vi "3_AdvancedDemo_TH260T3.vi"() -> ()   [LabVIEW 2010]
uses:
  Types/TH260_UIThread_Cmds.ctl
  Types/TH260_UIThread_Data.ctl
  Types/TH260_InputChannel.ctl
  <vilib>/Utility/error.llb/DialogType.ctl
  Types/TH260_DataProcThread_QCmds.ctl
  Types/TH260_DataProcThread_QData.ctl
  Types/TH260_VisThread_QCmds.ctl
  Types/TH260_VisThread_QData.ctl
  Types/TH260_VisThread_Data.ctl
  _lib/PQ/TimeHarp260/TH260_InitInfo.ctl
  _lib/PQ/TimeHarp260/th260lib_x86_x64_UIThread.llb/TH260_DllPath_global.vi
  _lib/PQ/TimeHarp260/TH260_LibVersion_global.vi
  _lib/PQ/TimeHarp260/TH260_MeasMode.ctl
  _lib/PQ/TimeHarp260/TH260_TimingMode.ctl
panel:
  in  "Settings":bool=TRUE
  in  "Run continuously":bool caption="Conti."
  in  "Start":bool
  in  "Scale":bool
  out "CountRates":i32[](graph)
  in  "HistoAcqTime":dbl=1.0 caption="Int.Time    s" min=0.1 max=360000.0 step=0.1
  in  "AcqTime":i32=360000000 caption="T3Acq.   ms" min=1 max=360000 step=1
  in  "Binning":i32(ring) caption="Resol.      ps" items=["250", "500", "1000", "2000", "4000", "8000", "16000", "32000", "64000", "128000", "256000", "512000", "1024000", "2048000", "4096000", "8192000", "16384000", "32768000", "65536000", "131072000", "262144000", "524288000"]
  in  "HistoOffset":i32 caption="Offset      ns" min=0 max=500000 step=1
  out "DeltaT":dbl=inf caption="Resol.     ms" format="%.2f"
  in  "BitShift":i32=15 min=0 max=32 step=1
  in  "OvlLevel":u32=65536 caption="Ovl.Level" min=1024 max=65536 step=1024
  in  "StopOvl.":bool=TRUE
  out "TTraceGraph":T1(graph)
  out "HistoGraph":cluster{dbl, "Resol":dbl, "Histos":u32[][]}(graph)
  in  "SyncTrgEdge":i32(ring) caption="Edge" items=["falling", "rising"]
  in  "SyncTrgLevel":i32=-100 caption="Level        mV" min=-1200 max=1200 step=1
  in  "SyncCFDLevel":i32=-100 caption="Level        mV" min=-1200 max=0 step=1
  in  "SyncZeroX":i32=-10 caption="ZeroCr.    mV" min=-40 max=0 step=1
  in  "SyncDivider":i32(ring)=3 caption="Divider" items=["1", "2", "4", "8"]
  in  "SyncOffset":i32 caption="Offset        ps" min=-99999 max=99999 step=1
  in  "Channels":T2[](array[typedef])=[{"Name"="Inp.Chan 1", "Enable"=TRUE, "Offset"=0, "CFDLevel"=50, "ZeroX"=10, "dtcode"=0, "TrgLevel"=-100, "TrgEdge"=0}, {"Name"="Inp.Chan 2", "Enable"=TRUE, "Offset"=0, "CFDLevel"=50, "ZeroX"=10, "dtcode"=0, "TrgLevel"=-100, "TrgEdge"=0}, {"Name"="Inp.Chan 3", "Enable"=TRUE, "Offset"=0, "CFDLevel"=50, "ZeroX"=10, "dtcode"=0, "TrgLevel"=-100, "TrgEdge"=0}, {"Name"="Inp.Chan 4", "Enable"=TRUE, "Offset"=0, "CFDLevel"=50, "ZeroX"=10, "dtcode"=0, "TrgLevel"=-100, "TrgEdge"=0}, {"Name"="Inp.Chan 5", "Enable"=TRUE, "Offset"=0, "CFDLevel"=50, "ZeroX"=10, "dtcode"=0, "TrgLevel"=-100, "TrgEdge"=0}, {"Name"="Inp.Chan 6", "Enable"=TRUE, "Offset"=0, "CFDLevel"=50, "ZeroX"=10, "dtcode"=0, "TrgLevel"=-100, "TrgEdge"=0}, {"Name"="Inp.Chan 7", "Enable"=TRUE, "Offset"=0, "CFDLevel"=50, "ZeroX"=10, "dtcode"=0, "TrgLevel"=-100, "TrgEdge"=0}, {"Name"="Inp.Chan 8", "Enable"=TRUE, "Offset"=0, "CFDLevel"=50, "ZeroX"=10, "dtcode"=0, "TrgLevel"=-100, "TrgEdge"=0}] {"TrgEdge" items=["falling", "rising"]; "TrgLevel" min=-1200 max=1200 step=1; "dtcode" items=["24", "44", "66", "88", "112", "135", "160", "180"]; "ZeroX" min=-40 max=0 step=1; "Offset" min=-99999 max=99999 step=1; "CFDLevel" min=-1200 max=0 step=1}
  out "SyncRate":string="Sync Rate: 0 cps\n"
  out "OverRun":bool caption="Overrun:"
  out "Status":string="Elements in Q: 0"
  # "Histogram"
  # "Time Trace"
  # "Sync"
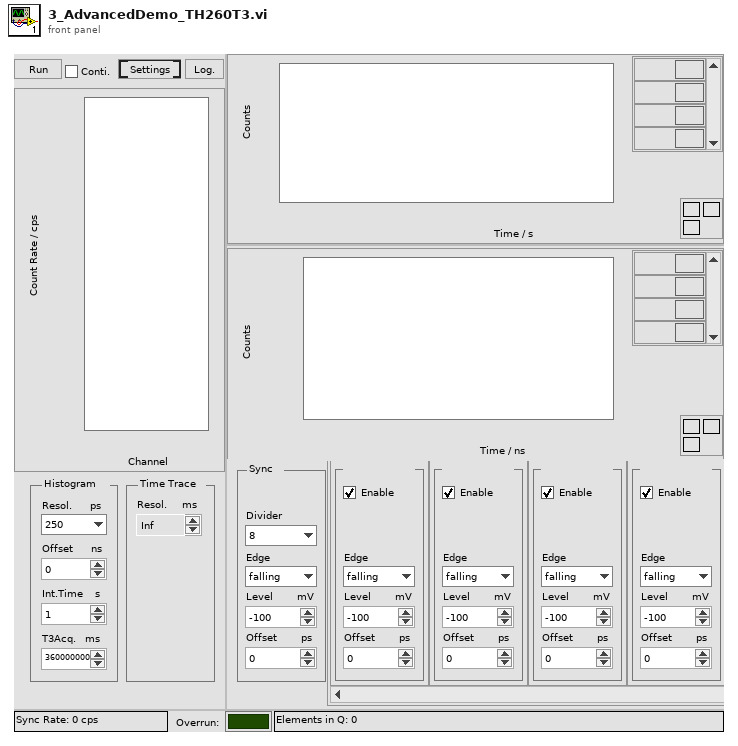
[diagram p1: front panel]
types:
  T1 = cluster{dbl, "Resolution":dbl, "Histogram":u32[][]}
  T2 = typedef "TH260_InputChannel.ctl" = cluster{"Name":string, "Enable":bool, "Offset":i32, "CFDLevel":i32, "ZeroX":i32, "dtcode":i32, "TrgLevel":i32, "TrgEdge":i32}
  T3 = typedef "TH260_DataProcThread_QCmds.ctl" = enum16{"Exit", "Proc", "Init", "SetShift", "SetNumChannels", "SetHistAcqTime"}
  T4 = typedef "TH260_VisThread_Data.ctl" = cluster{"Resol":dbl, "DeltaT":dbl, "NumChannels":i32}
  T5 = typedef "TH260_VisThread_QData.ctl" = cluster{"Histos":u32[][], "Cmd":T6, "TimeTrace":u32[][], "Bin":i32, "Total bin":u64, "Status":string, "Resol":dbl, "DeltaT":dbl, "nChannels":i32}
  T6 = typedef "TH260_VisThread_QCmds.ctl" = enum16{"_none_", "Resol", "nChannels", "DeltaT", "Histo", "TTrace", "Status"}
  T7 = typedef "TH260_DataProcThread_QData.ctl" = cluster{"Cmd":T3, "nActual":i32, "Buffer":u32[], "TickCount":u32, "Param":i32}
  T8 = typedef "TH260_UIThread_Data.ctl" = cluster{"Init Info":T9, "DevIdx":i32, "Channels":T2[], "CurrentChannels":i32[], "AcqTime":i32, "Binning":i32, "HistoOffset":i32, "HistoLen":i32, "StopOvl.":bool, "OvlLevel":u32, "StartMeas":bool, "HistoLength":i32, "Resolution":dbl, "Run cont.":bool, "Status":string, "SyncRate":i32, "BitShift":i32, "HistoAcqTime":dbl, "SyncTrgEdge":i32, "SyncTrgLevel":i32, "SyncCFDLevel":i32, "SyncZeroX":i32, "SyncDivider":i32, "SyncOffset":i32}
  T9 = typedef "TH260_InitInfo.ctl" = cluster{"Library Version":string, "Serial No.":string, "Model":string, "Partnum":string, "Version":string, "features":i32, "nchannels":i32, "Base Resolution":dbl, "Bin Steps":i32}
  T10 = typedef "TH260_UIThread_Cmds.ctl" = enum16{"Idle", "Init", "SetInpChanEnable", "SetInpChanOffset", "SetInpChanCFD", "SetInpChanTrg", "SetInpChanDeadtime", "SetSyncDivider", "SetSyncCFD", "SetSyncTrg", "SetSyncOffset", "SetBinning", "SetHistoOffset", "SetHistoLen", "SetStopOvl", "SetBitShift", "SetHistoAcqTime", "GetRates", "StartMeas", "StopMeas", "AbortMeas", "GetResolution", "GetHisto", "ReadFiFo", "WriteStatus", "Resize", "EnableControls", "DisableControls", "Error", "Exit"}
  T11 = enum8{"Enabled", "Disabled", "Disabled and Grayed Out"}
  T12 = typedef "TH260_TimingMode.ctl" = i32
  T13 = typedef "TH260_MeasMode.ctl" = i32
  T14 = typedef "DialogType.ctl" = u16
  T15 = cluster{"T0":dbl, "dt":dbl, "TimeTrace_out":u32[][]}
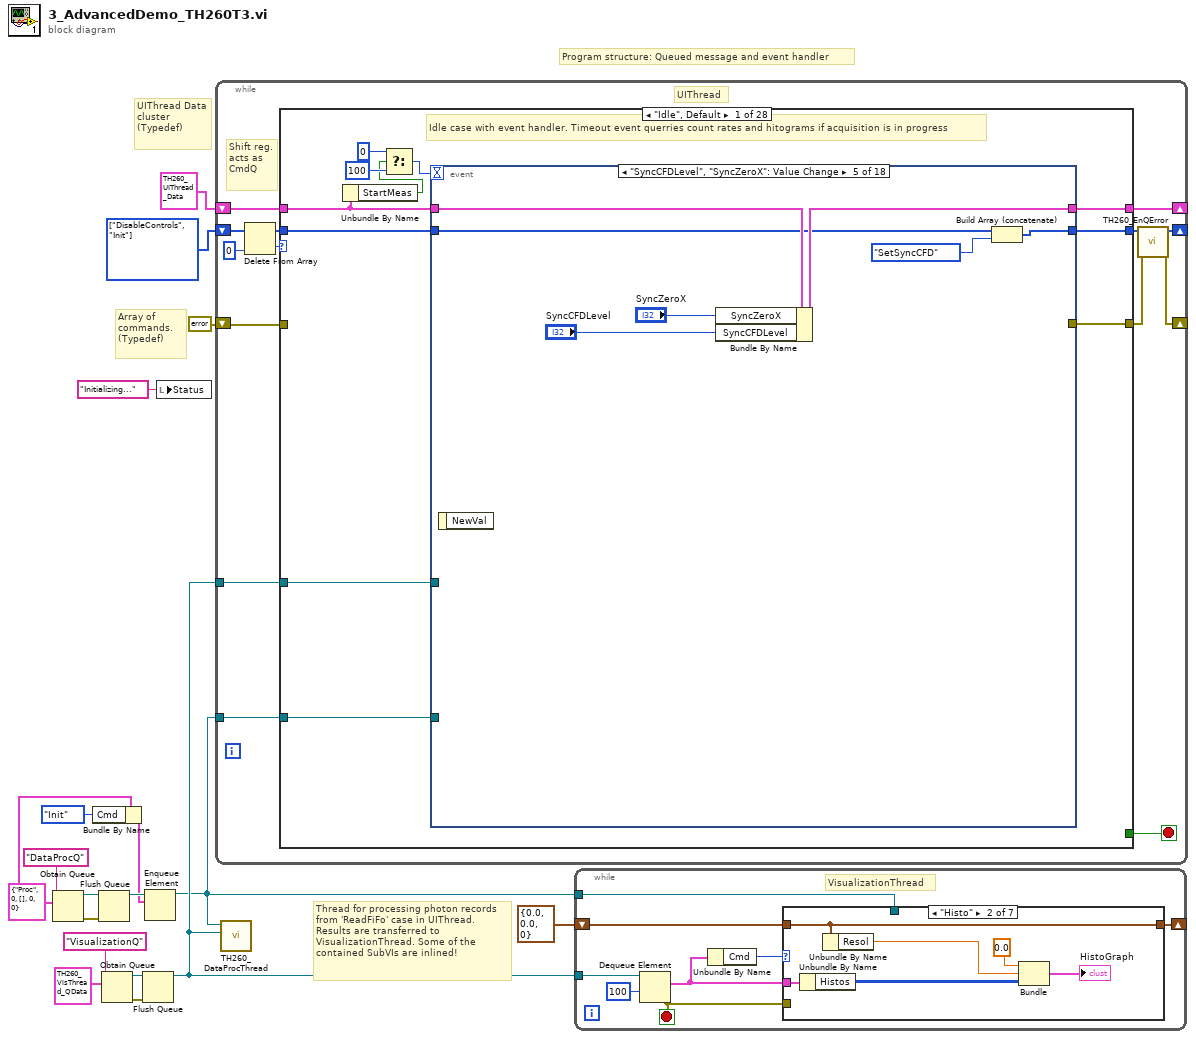
[diagram p0: block diagram]
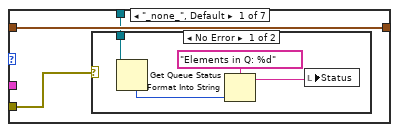
[diagram p2: hidden frame]
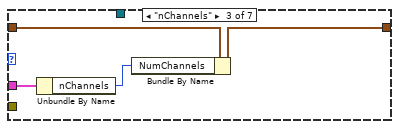
[diagram p4: hidden frame]
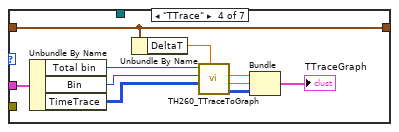
[diagram p5: hidden frame]
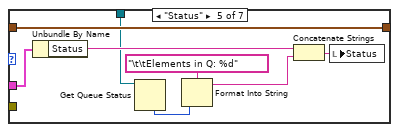
[diagram p6: hidden frame]
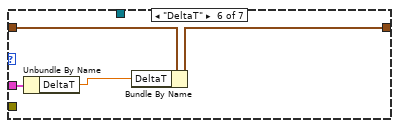
[diagram p7: hidden frame]
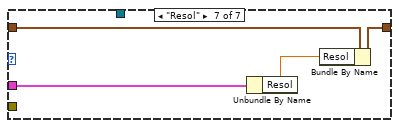
[diagram p8: hidden frame]
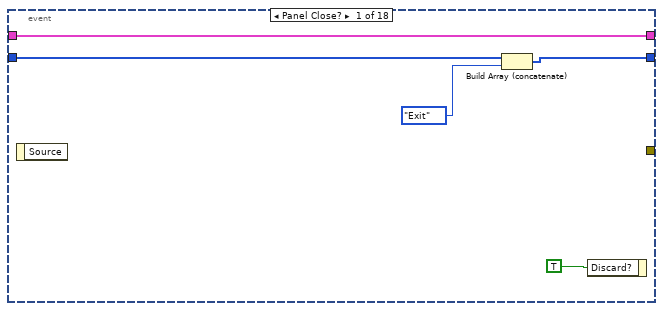
[diagram p9: hidden frame]
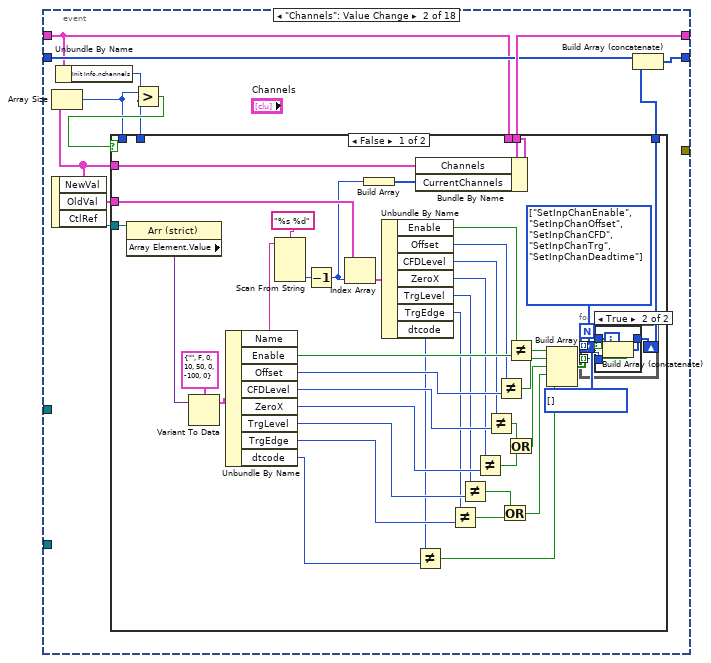
[diagram p10: hidden frame]
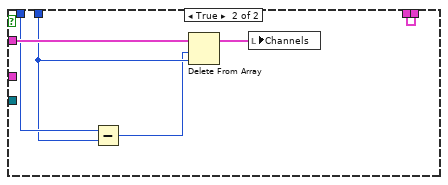
[diagram p12: hidden frame]
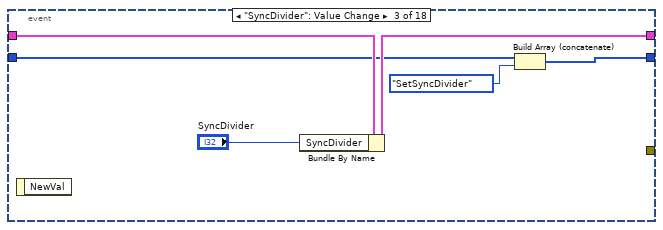
[diagram p13: hidden frame]
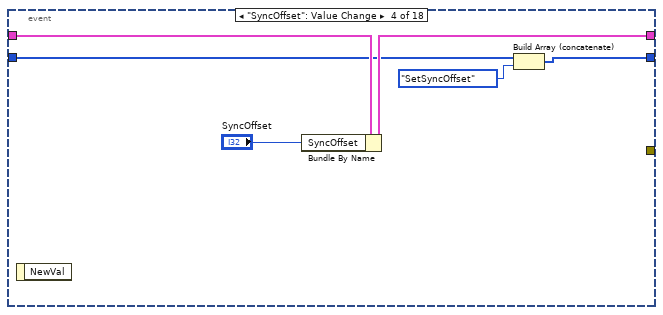
[diagram p14: hidden frame]
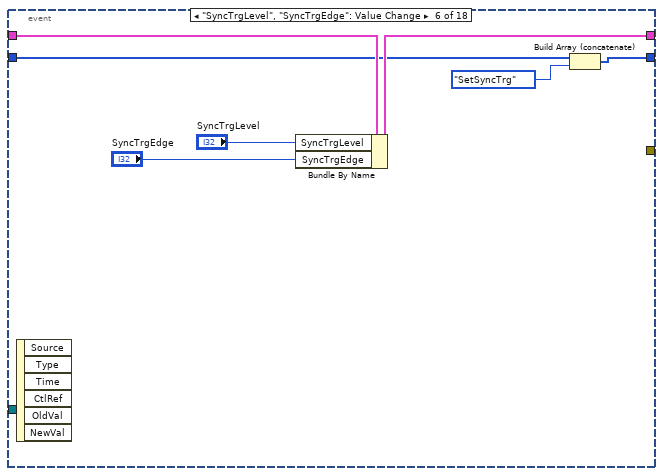
[diagram p15: hidden frame]
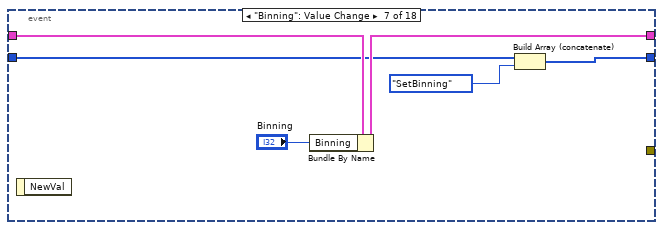
[diagram p16: hidden frame]
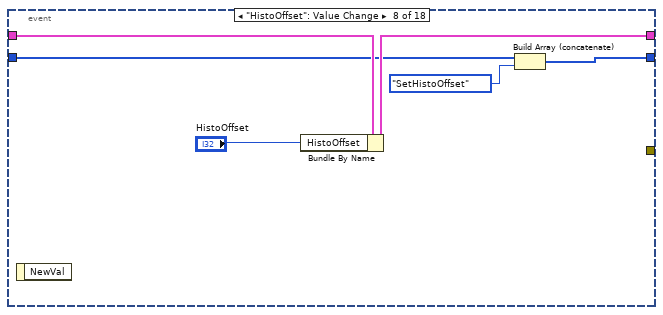
[diagram p17: hidden frame]
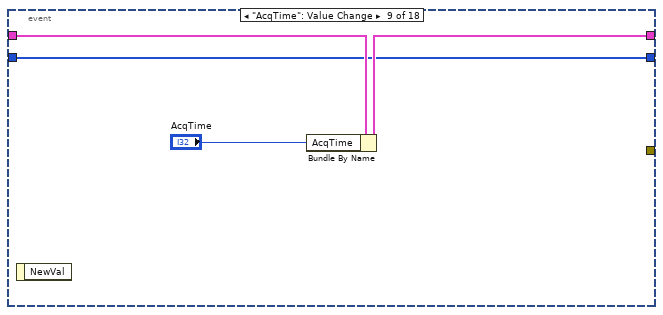
[diagram p18: hidden frame]
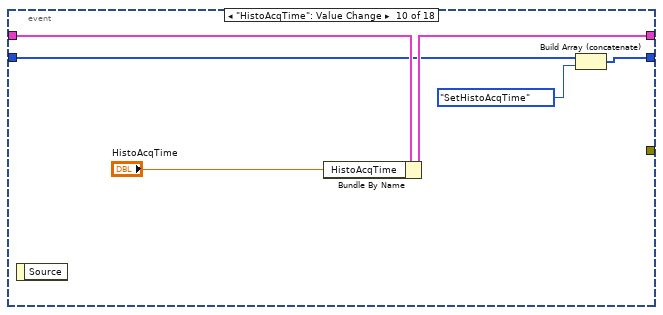
[diagram p19: hidden frame]
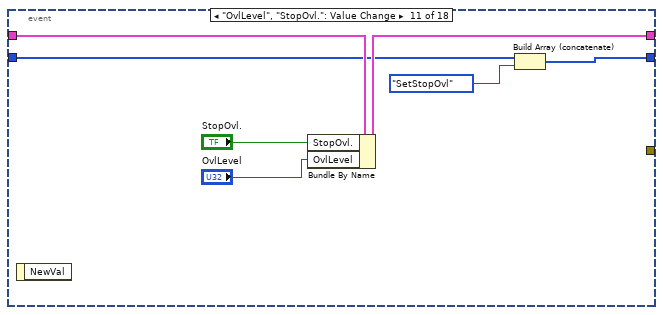
[diagram p20: hidden frame]
diagram:
  w4 = T7 {"Cmd"=enum."Proc", "nActual"=0, "Buffer"=[], "TickCount"=0, "Param"=0} ("MH_DataProcThread_QData")
  w17 = T10[] [enum."DisableControls", enum."Init"] items=["Idle", "Init", "SetInpChanEnable", "SetInpChanOffset", "SetInpChanCFD", "SetInpChanTrg", "SetInpChanDeadtime", "SetSyncDivider", "SetSyncCFD", "SetSyncTrg", "SetSyncOffset", "SetBinning", "SetHistoOffset", "SetHistoLen", "SetStopOvl", "SetBitShift", "SetHistoAcqTime", "GetRates", "StartMeas", "StopMeas", "AbortMeas", "GetResolution", "GetHisto", "ReadFiFo", "WriteStatus", "Resize", "EnableControls", "DisableControls", "Error", "Exit"]
  # "Thread for processing photon records from 'ReadFiFo' case in UIThread. Results are transferred to VisualizationThread. Some of the contained SubVIs are inlined!"
  # "Array of commands.\n(Typedef)"
  # "Program structure: Queued message and event handler"
  # "UIThread Data cluster\n(Typedef)"
  n1 = Obtain Queue(name (unnamed)="DataProcQ", element data type=w4) -> (queue out=w14:refnum<queue>, error out=w13:errorcluster)  [unwired: 3 in, 1 out]
  n2 = Bundle By Name(cluster=w4, "Cmd"=TH260_DataProcThread_QCmds."Init") -> (w2:T7)
  n3 = Flush Queue(queue=w14, error in (no error)=w13) -> (queue out=w5:refnum<queue>)  [unwired: 2 out]
  n4 = Obtain Queue(name (unnamed)="VisualizationQ", element data type=T5 {"Histos"=[], "Cmd"=enum."_none_", "TimeTrace"=[], "Bin"=0, "Total bin"=0, "Status"="", "Resol"=0.0, "DeltaT"=0.0, "nChannels"=0} ("MH_GUIThread_QData")) -> (queue out=w12:refnum<queue>, error out=w11:errorcluster)  [unwired: 3 in, 1 out]
  n5 = Flush Queue(queue=w12, error in (no error)=w11) -> (queue out=w7:refnum<queue>)  [unwired: 2 out]
  n6 = Enqueue Element(queue=w5, element=w2) -> (queue out=w1:refnum<queue>)  [unwired: 2 in, 2 out]
  n7 = local write "Status"("Initializing..." ("Status")) -> ()
  n8 = while {
    shift-right: [w21] -> _
    shift-left: w17 -> [w28]
    shift-right: [w31] -> _
    shift-left: T8 {"Init Info"={"Library Version"="", "Serial No."="", "Model"="", "Partnum"="", "Version"="", "features"=0, "nchannels"=0, "Base Resolution"=0.0, "Bin Steps"=0}, "DevIdx"=0, "Channels"=[], "CurrentChannels"=[], "AcqTime"=1, "Binning"=1, "HistoOffset"=1, "HistoLen"=1024, "StopOvl."=FALSE, "OvlLevel"=1024, "StartMeas"=FALSE, "HistoLength"=0, "Resolution"=0.0, "Run cont."=FALSE, "Status"="", "SyncRate"=0, "BitShift"=0, "HistoAcqTime"=0.0, "SyncTrgEdge"=50, "SyncTrgLevel"=0, "SyncCFDLevel"=-100, "SyncZeroX"=10, "SyncDivider"=1, "SyncOffset"=0} -> [w30]
    shift-right: [w23] -> _
    shift-left: errorcluster {"status"=FALSE, "code"=0, "source"=""} ("error IO") -> [w29]
    tunnel: w1 -> [w20]
    tunnel: w7 -> [w19]
    stop <- w32 stop-if-true
    # "Shift reg.\nacts as\nCmdQ"
    # "UIThread"
    n9 = Delete From Array(array=w28, index=0) -> (deleted portion=w26:T10, array with subset deleted=w25:T10[])  [unwired: 1 in]
    n10 = case shown="\"Idle\", Default" w26 {
      tunnel: [w43 w308 w337 w351 w365 w380 w395 w411 w420 w426 w428 w435 w443 w449 w469 w481 w493 w513 w519 w532 w549 w550 w576 w589 w596 w608 w614 w620] -> w22
      tunnel: [_ _ _ _ _ _ _ _ _ _ _ _ _ _ _ _ _ _ _ _ _ _ _ _ _ _ _ TRUE] -> w32
      tunnel: [w42 w289 w340 w354 w368 w383 w398 w413 w421 w427 w432 w439 w444 w450 w454 w471 w483 w517 w522 w534 w545 w560 w575 w577 w595 w607 w615 w623] -> w31
      tunnel: w30 -> [w39 w294 w340 w354 w368 w383 w398 w413 w421 w427 w432 w439 w444 w450 w454 w471 w484 w517 w523 w535 w546 w560 w575 w577 w595 w607 w615 w623]
      tunnel: [w40 w312 w338 w352 w366 w381 w396 w409 w419 w425 w431 w438 w442 w448 _ _ w492 w516 w525 w537 w547 w555 _ _ _ _ _ w621] -> w24
      tunnel: w29 -> [_ _ _ _ _ _ _ _ _ _ _ _ _ _ _ _ _ _ _ _ _ _ _ _ _ _ w616 _]
      tunnel: w25 -> [w41 w309 w337 w351 w365 w380 w395 w411 w420 w426 w428 w434 w443 w449 w469 w481 w493 w514 w520 w532 w549 w551 w576 w589 w596 w608 _ w620]
      tunnel: w20 -> [w34 w287 _ _ _ _ _ _ _ _ _ _ _ _ w455 w472 _ w510 _ _ _ w552 _ _ _ _ _ w619]
      tunnel: w19 -> [w33 w279 _ _ _ _ _ _ _ _ _ _ _ _ w456 _ _ _ _ _ w542 _ _ _ _ _ _ w618]
      frame "Idle", Default {
        # "Idle case with event handler. Timeout event querries count rates and hitograms if acquisition is in progress"
        n11 = Unbundle By Name(w39) -> ("StartMeas"=w37:bool)
        n12 = Select(t=0, s=w37, f=100) -> (s? t:f=w36:i32)
        n13 = event shown="[4] \"SyncCFDLevel\", \"SyncZeroX\": Value Change" {
          selector: _ -> [_ _ _ _ _ _ _ _ _ _ _ _ _ _ _ _ _ _]
          dyn-events: _ -> [_ _ _ _ _ _ _ _ _ _ _ _ _ _ _ _ _ _]
          timeout: w36 -> [_ _ _ _ _ _ _ _ _ _ _ _ _ _ _ _ _ _]
          tunnel: [w44 w54 w116 w122 w129 w136 w142 w148 w153 w158 w165 w180 w198 w210 w228 w234 w242 w252] -> w43
          tunnel: [w47 w57 w119 w125 w132 w139 w145 w151 w155 w161 w168 w179 w202 w209 w226 w233 w241 w255] -> w42
          tunnel: w39 -> [w47 w53 w120 w126 w133 w140 w146 w152 w156 w162 w169 w179 w203 w207 w227 w233 w241 w255]
          tunnel: w41 -> [w46 w56 w118 w124 w131 w138 w144 w150 w153 w159 w167 w181 w199 w211 w228 w234 w242 w253]
          tunnel: [_ _ _ _ _ _ _ _ _ _ _ w175 _ _ _ _ _ _] -> w40
          tunnel: w34 -> [_ _ _ _ _ _ _ _ _ _ _ _ _ _ _ _ _ _]
          tunnel: w33 -> [_ _ _ _ _ _ _ _ _ _ _ _ _ _ _ _ _ _]
          event Panel Close? {
            n14 = event-data() -> ()  [unwired: 1 in, 1 out]
            n15 = Build Array (concatenate)(w46, TH260_UIThread_Cmds."Exit") -> (w44:T10[])
            n16 = event-data("Discard?"=TRUE) -> ()  [unwired: 1 in, 1 out]
          }
          event "Channels": Value Change {
            n17 = event-data() -> ("NewVal"=w52:T2[], "OldVal"=w58:T2[], "CtlRef"=w59:refnum<vi>)  [unwired: 1 in]
            n18 = Array Size(array=w52) -> (size(s)=w49:i32)
            n19 = Unbundle By Name(w53) -> ("Init Info.nchannels"=w50:i32)
            n20 = Greater?(x=w49, y=w50) -> (0:w51:bool)
            n21 = case shown="False" w51 {
              tunnel: w59 -> [w100 _]
              tunnel: w58 -> [w94 _]
              tunnel: [w77 w114] -> w57
              tunnel: [w75 _] -> w55
              tunnel: w53 -> [w72 w114]
              tunnel: w52 -> [w71 w113]
              tunnel: w50 -> [_ w111]
              tunnel: w49 -> [_ w112]
              frame False {
                w60 = T10[] [] items=["Idle", "Init", "SetInpChanEnable", "SetInpChanOffset", "SetInpChanCFD", "SetInpChanTrg", "SetInpChanDeadtime", "SetSyncDivider", "SetSyncCFD", "SetSyncTrg", "SetSyncOffset", "SetBinning", "SetHistoOffset", "SetHistoLen", "SetStopOvl", "SetBitShift", "SetHistoAcqTime", "GetRates", "StartMeas", "StopMeas", "AbortMeas", "GetResolution", "GetHisto", "ReadFiFo", "WriteStatus", "Resize", "EnableControls", "DisableControls", "Error", "Exit"] ("Array")
                w78 = T10[] [enum."SetInpChanEnable", enum."SetInpChanOffset", enum."SetInpChanCFD", enum."SetInpChanTrg", enum."SetInpChanDeadtime"] items=["Idle", "Init", "SetInpChanEnable", "SetInpChanOffset", "SetInpChanCFD", "SetInpChanTrg", "SetInpChanDeadtime", "SetSyncDivider", "SetSyncCFD", "SetSyncTrg", "SetSyncOffset", "SetBinning", "SetHistoOffset", "SetHistoLen", "SetStopOvl", "SetBitShift", "SetHistoAcqTime", "GetRates", "StartMeas", "StopMeas", "AbortMeas", "GetResolution", "GetHisto", "ReadFiFo", "WriteStatus", "Resize", "EnableControls", "DisableControls", "Error", "Exit"]
                n22 = property class="Arr (strict)"(reference=w100) -> ("Array Element.Value"=w99:variant)  [unwired: 1 in, 2 out]
                n23 = Variant To Data(Variant=w99, type=T2 {"Name"="", "Enable"=FALSE, "Offset"=0, "CFDLevel"=10, "ZeroX"=50, "dtcode"=0, "TrgLevel"=-100, "TrgEdge"=0} ("Channel")) -> (data=w76:cluster{})  [unwired: 1 in, 1 out]
                n24 = Unbundle By Name(w76) -> ("Name"=w97:string, "Enable"=w91:bool, "Offset"=w89:i32, "CFDLevel"=w87:i32, "ZeroX"=w85:i32, "TrgLevel"=w69:i32, "TrgEdge"=w67:i32, "dtcode"=w62:i32)
                n25 = Scan From String(format string="%s %d", input string=w97) -> (output 2=w95:i32)  [unwired: 5 in, 3 out]
                n26 = Decrement(x=w95) -> (x-1=w74:i32)
                n27 = Index Array(array=w94, index=w74) -> (element=w93:T2)
                n28 = Build Array(w74) -> (w73:i32[])
                n29 = Unbundle By Name(w93) -> ("Enable"=w92:bool, "Offset"=w90:i32, "CFDLevel"=w88:i32, "ZeroX"=w86:i32, "TrgLevel"=w70:i32, "TrgEdge"=w68:i32, "dtcode"=w63:i32)
                n30 = Not Equal?(x=w63, y=w62) -> (x != y?=w61:bool)
                n31 = Bundle By Name(cluster=w72, "Channels"=w71, "CurrentChannels"=w73) -> (w77:T8)
                n32 = Not Equal?(x=w68, y=w67) -> (x != y?=w65:bool)
                n33 = Not Equal?(x=w70, y=w69) -> (x != y?=w66:bool)
                n34 = Not Equal?(x=w86, y=w85) -> (x != y?=w80:bool)
                n35 = Not Equal?(x=w88, y=w87) -> (x != y?=w81:bool)
                n36 = Not Equal?(x=w90, y=w89) -> (x != y?=w83:bool)
                n37 = Or(x=w66, y=w65) -> (x .or. y?=w64:bool)
                n38 = Not Equal?(x=w92, y=w91) -> (x != y?=w84:bool)
                n39 = Or(x=w81, y=w80) -> (x .or. y?=w79:bool)
                n40 = Build Array(w84, w83, w79, w64, w61) -> (w82:bool[])
                n41 = for {
                  tunnel: w82 -> [w103] mode=indexing
                  tunnel: w78 -> [w104] mode=indexing
                  shift-right: [w101] -> w75
                  shift-left: w60 -> [w102]
                  n42 = case shown="True" w103 {
                    tunnel: w102 -> [w105 w107]
                    tunnel: w104 -> [_ w106]
                    tunnel: [w105 w108] -> w101
                    frame False {
                    }
                    frame True {
                      n43 = Build Array (concatenate)(w107, w106) -> (w108:T10[])
                    }
                  }
                }
              }
              frame True {
                n44 = Subtract(x=w112, y=w111) -> (x-y=w110:i32)
                n45 = Delete From Array(array=w113, length=w110, index=w111) -> (array with subset deleted=w109:T2[])  [unwired: 1 out]
                n46 = local write "Channels"(w109) -> ()
              }
            }
            n47 = Build Array (concatenate)(w56, w55) -> (w54:T10[])
          }
          event "SyncDivider": Value Change {
            n48 = event-data() -> ()  [unwired: 1 in, 1 out]
            n49 = Bundle By Name(cluster=w120, "SyncDivider"="SyncDivider") -> (w119:T8)
            n50 = Build Array (concatenate)(w118, TH260_UIThread_Cmds."SetSyncDivider") -> (w116:T10[])
          }
          event "SyncOffset": Value Change {
            n51 = event-data() -> ()  [unwired: 1 in, 1 out]
            n52 = Bundle By Name(cluster=w126, "SyncOffset"="SyncOffset") -> (w125:T8)
            n53 = Build Array (concatenate)(w124, TH260_UIThread_Cmds."SetSyncOffset") -> (w122:T10[])
          }
          event "SyncCFDLevel", "SyncZeroX": Value Change {
            n54 = event-data() -> ()  [unwired: 1 in, 1 out]
            n55 = Bundle By Name(cluster=w133, "SyncZeroX"="SyncZeroX", "SyncCFDLevel"="SyncCFDLevel") -> (w132:T8)
            n56 = Build Array (concatenate)(w131, TH260_UIThread_Cmds."SetSyncCFD") -> (w129:T10[])
          }
          event "SyncTrgLevel", "SyncTrgEdge": Value Change {
            n57 = event-data() -> ()  [unwired: 1 in, 6 out]
            n58 = Bundle By Name(cluster=w140, "SyncTrgLevel"="SyncTrgLevel", "SyncTrgEdge"="SyncTrgEdge") -> (w139:T8)
            n59 = Build Array (concatenate)(w138, TH260_UIThread_Cmds."SetSyncTrg") -> (w136:T10[])
          }
          event "Binning": Value Change {
            n60 = event-data() -> ()  [unwired: 1 in, 1 out]
            n61 = Bundle By Name(cluster=w146, "Binning"="Binning") -> (w145:T8)
            n62 = Build Array (concatenate)(w144, TH260_UIThread_Cmds."SetBinning") -> (w142:T10[])
          }
          event "HistoOffset": Value Change {
            n63 = event-data() -> ()  [unwired: 1 in, 1 out]
            n64 = Bundle By Name(cluster=w152, "HistoOffset"="HistoOffset") -> (w151:T8)
            n65 = Build Array (concatenate)(w150, TH260_UIThread_Cmds."SetHistoOffset") -> (w148:T10[])
          }
          event "AcqTime": Value Change {
            n66 = event-data() -> ()  [unwired: 1 in, 1 out]
            n67 = Bundle By Name(cluster=w156, "AcqTime"="AcqTime") -> (w155:T8)
          }
          event "HistoAcqTime": Value Change {
            n68 = event-data() -> ()  [unwired: 1 in, 1 out]
            n69 = Bundle By Name(cluster=w162, "HistoAcqTime"="HistoAcqTime") -> (w161:T8)
            n70 = Build Array (concatenate)(w159, TH260_UIThread_Cmds."SetHistoAcqTime") -> (w158:T10[])
          }
          event "OvlLevel", "StopOvl.": Value Change {
            n71 = event-data() -> ()  [unwired: 1 in, 1 out]
            n72 = Bundle By Name(cluster=w169, "StopOvl."="StopOvl.", "OvlLevel"="OvlLevel") -> (w168:T8)
            n73 = Build Array (concatenate)(w167, TH260_UIThread_Cmds."SetStopOvl") -> (w165:T10[])
          }
          event Timeout {
            n74 = event-data() -> ()  [unwired: 1 in, 1 out]
            n75 = Unbundle By Name(w179) -> ("DevIdx"=w177:i32, "StartMeas"=w178:bool, "BitShift"=w174:i32, "SyncRate"=w173:i32)
            n76 = case shown="True" w178 {
              tunnel: w177 -> [_ w197]
              tunnel: [_ w195] -> w176
              tunnel: [_ w192] -> w175
              frame False {
              }
              frame True {
                w193 = T10[] [enum."ReadFiFo"] items=["Idle", "Init", "SetInpChanEnable", "SetInpChanOffset", "SetInpChanCFD", "SetInpChanTrg", "SetInpChanDeadtime", "SetSyncDivider", "SetSyncCFD", "SetSyncTrg", "SetSyncOffset", "SetBinning", "SetHistoOffset", "SetHistoLen", "SetStopOvl", "SetBitShift", "SetHistoAcqTime", "GetRates", "StartMeas", "StopMeas", "AbortMeas", "GetResolution", "GetHisto", "ReadFiFo", "WriteStatus", "Resize", "EnableControls", "DisableControls", "Error", "Exit"]
                w194 = T10[] [enum."StopMeas"] items=["Idle", "Init", "SetInpChanEnable", "SetInpChanOffset", "SetInpChanCFD", "SetInpChanTrg", "SetInpChanDeadtime", "SetSyncDivider", "SetSyncCFD", "SetSyncTrg", "SetSyncOffset", "SetBinning", "SetHistoOffset", "SetHistoLen", "SetStopOvl", "SetBitShift", "SetHistoAcqTime", "GetRates", "StartMeas", "StopMeas", "AbortMeas", "GetResolution", "GetHisto", "ReadFiFo", "WriteStatus", "Resize", "EnableControls", "DisableControls", "Error", "Exit"]
                n77 = call "TH260_CTCStatus.vi"("devidx"=w197) -> ("error out"=w192:errorcluster, "ctcstatus"=w196:i32)  [unwired: 8 in, 1 out]
                n78 = Not Equal To 0?(x=w196) -> (x != 0?=w191:bool)
                n79 = Select(t=w194, s=w191, f=w193) -> (s? t:f=w195:T10[])
              }
            }
            n80 = call "CalcRate.vi"("Refresh(ms)"=u32 100) -> ("updated?"=w171:bool)  [unwired: 8 in, 2 out]
            n81 = case shown="True" w171 {
              tunnel: w174 -> [_ w184]
              tunnel: w173 -> [_ w183]
              tunnel: [_ TH260_UIThread_Cmds."GetRates"] -> w172
              frame False {
              }
              frame True {
                n82 = To Double Precision Float(number=w183) -> (double precision float=w188:dbl)
                n83 = To Double Precision Float(number=w184) -> (double precision float=w189:dbl)
                n84 = Power Of 2(x=w189) -> (2^x=w187:dbl)
                n85 = Multiply(x=w187, y=1000.0) -> (x*y=w186:dbl)
                n86 = Divide(x=w186, y=w188) -> (x/y=w190:dbl)
                n87 = local write "DeltaT"(w190) -> ()
              }
            }
            n88 = Build Array (concatenate)(w181, w176, w172) -> (w180:T10[])
          }
          event "BitShift": Value Change {
            n89 = event-data() -> ()  [unwired: 1 in, 1 out]
            n90 = Bundle By Name(cluster=w203, "BitShift"="BitShift") -> (w202:T8)
            n91 = Build Array (concatenate)(w199, TH260_UIThread_Cmds."SetBitShift") -> (w198:T10[])
          }
          event "Start": Value Change {
            n92 = event-data() -> ()  [unwired: 1 in, 1 out]
            n93 = Unbundle By Name(w207) -> ("SyncRate"=w206:i32)
            n94 = Greater Or Equal?(x=w206, y=10) -> (x >= y?=w204:bool)
            n95 = case shown="True" w204 {
              selector: w204 -> [w213 _]
              tunnel: w211 -> [w215 w224]
              tunnel: [w215 w222] -> w210
              tunnel: [w214 w221] -> w209
              tunnel: "Start" -> [_ w220]
              tunnel: w207 -> [w214 w216]
              frame False {
                n96 = local write "Start"(w213) -> ()
                n97 = One Button Dialog(message="SyncRate too low!!!" ("Status")) -> ()  [unwired: 1 in, 1 out]
              }
              frame True {
                w219 = T10[] [enum."SetBitShift", enum."SetHistoAcqTime", enum."StartMeas"] items=["Idle", "Init", "SetInpChanEnable", "SetInpChanOffset", "SetInpChanCFD", "SetInpChanTrg", "SetInpChanDeadtime", "SetSyncDivider", "SetSyncCFD", "SetSyncTrg", "SetSyncOffset", "SetBinning", "SetHistoOffset", "SetHistoLen", "SetStopOvl", "SetBitShift", "SetHistoAcqTime", "GetRates", "StartMeas", "StopMeas", "AbortMeas", "GetResolution", "GetHisto", "ReadFiFo", "WriteStatus", "Resize", "EnableControls", "DisableControls", "Error", "Exit"]
                n98 = Bundle By Name(cluster=w216, "StartMeas"=w220) -> (w221:T8)
                n99 = Build Array(TH260_UIThread_Cmds."AbortMeas") -> (w217:T10[])
                n100 = Select(t=w219, s=w220, f=w217) -> (s? t:f=w223:T10[])
                n101 = Build Array (concatenate)(w224, w223) -> (w222:T10[])
              }
            }
          }
          event "Run continuously": Value Change {
            n102 = event-data() -> ()  [unwired: 1 in, 1 out]
            n103 = Bundle By Name(cluster=w227, "Run cont."="Run continuously") -> (w226:T8)
          }
          event "Scale": Value Change {
            n104 = event-data() -> ()  [unwired: 1 in, 1 out]
            n105 = Select(t=u8 0 ("Y Scale.Mapping Mode"), s="Scale", f=u8 1 ("Y Scale.Mapping Mode")) -> (s? t:f=w229:u8)
            n106 = property on="HistoGraph" class="WFGraph (strict)"("YScale.Mapping Mode"=w229) -> ()  [unwired: 2 in, 2 out]
          }
          event "Settings": Value Change {
            n107 = event-data() -> ()  [unwired: 1 in, 1 out]
            n108 = property on="Splitter" class="Splitter"() -> ("Position"=w240:i32)  [unwired: 2 in, 2 out]
            n109 = Select(t=250 ("PosT"), s="Settings", f=0 ("PosF")) -> (s? t:f=w237:i32)
            n110 = Subtract(x=w240, y=w237) -> (x-y=w236:i32)
            n111 = while {
              shift-right: [w251] -> _
              shift-left: w236 -> [w244]
              i -> [w250]
              stop <- w247 stop-if-true
              n112 = property on="Splitter 4" class="Splitter"("Position"=w244) -> (error out=w243:errorcluster)  [unwired: 2 in, 1 out]
              n113 = Greater Or Equal?(x=w250, y=10) -> (x >= y?=w248:bool)
              n114 = Decrement(x=w244) -> (x-1=w251:i32)
              n115 = Unbundle(w243) -> ("status"=w246:bool)  [unwired: 2 out]
              n116 = Not(x=w246) -> (.not. x?=w245:bool)
              n117 = Or(x=w245, y=w248) -> (x .or. y?=w247:bool)
            }
          }
          event Panel Resize {
            n118 = event-data() -> ()  [unwired: 1 in, 1 out]
            n119 = Build Array (concatenate)(w253, TH260_UIThread_Cmds."Resize") -> (w252:T10[])
          }
        }
      }
      frame "Init" {
        w265 = -100 ("SyncTrgLevel")
        w266 = 0 ("SyncTrgEdge")
        w268 = T12 0 items=["Hires", "Lowres"]  # TimingMode
        w269 = T13 3 items=["Histo"=0, "T2"=2, "T3"=3]  # MeasMode
        w277 = 1.0 ("HistoAcqTime")
        w278 = 15 ("Value (Signaling)")
        w296 = FALSE ("Run cont.")
        w298 = FALSE ("StartMeas")
        w299 = u32 100000 ("OvlLevel")
        w300 = TRUE ("StopOvl.")
        w301 = 360000000 ("AcqTime")
        w302 = 0 ("HistoOffset")
        w303 = 0 ("Binning")
        w304 = -100 ("SyncLevel")
        w305 = -10 ("SyncZeroX")
        w306 = 0 ("SyncOffset")
        w307 = 3 ("SyncDivider")
        # "100 x 60 x 60 x 1000 = 100 h"
        # "Init all FP controls and corresponding copy in UIThread Data cluster"
        # "EnQ list of commands"
        # "Array with Inp.Chan."
        # "Initialization: 1. Init HW -> get # of channels -> make array for Inp.Channels\n2. Init all FP controls and corresponding fields in UIThread Data cluster\n3. EnQ list of commands for further initialization"
        n120 = call <vilib>:"Error Cluster From Error Code.vi"("is warning? (False)"=FALSE, "show call chain? (False)"=TRUE, "error message (\"\")"="DLL not found!" ("error message (\"\")"), "error code (0)"=5000) -> ("error out"=w271:errorcluster)  [unwired: 5 in]
        n121 = call "GetDLLPath.vi"("DllName_32bit"="TH260Lib.dll" ("name or relative path"), "DllName_64bit"="TH260Lib64.dll" ("name or relative path")) -> ("file exists?"=w273:bool, "DLLPath"=w274:path)  [unwired: 8 in]
        n122 = global write "TH260_DllPath_global.vi" "DllPath"(w274) -> ()
        n123 = Select(t=errorcluster {"status"=FALSE, "code"=0, "source"=""} ("error IO"), s=w273, f=w271) -> (s? t:f=w290:errorcluster)
        n124 = global read "TH260_LibVersion_global.vi" "Library Version"() -> (w270:string)
        n125 = property on="Settings" class="Bool (strict)"("Val(Sgnl)"=TRUE ("Value (Signaling)")) -> ()  [unwired: 2 in, 2 out]
        n126 = property on="Scale" class="Bool (strict)"("Val(Sgnl)"=FALSE ("Value (Signaling)")) -> ()  [unwired: 2 in, 2 out]
        n127 = call "InitTH260_UIThread.vi"("error in (no error)"=w290, "MeasMode"=w269, "TimingMode"=w268, "Library Version"=w270) -> ("error out"=w312:errorcluster, "Init Info"=w264:T9, "DevIdx"=w314:i32)  [unwired: 5 in]
        n128 = Unbundle By Name(w264) -> ("Model"=w263:string)
        n129 = local write "SyncDivider"(w307) -> ()
        n130 = local write "SyncOffset"(w306) -> ()
        n131 = local write "SyncZeroX"(w305) -> ()
        n132 = local write "SyncCFDLevel"(w304) -> ()
        n133 = local write "SyncTrgEdge"(w266) -> ()
        n134 = local write "SyncTrgLevel"(w265) -> ()
        n135 = Bundle By Name(cluster=w294, "DevIdx"=w314, "Status"="Initialized!", "Init Info"=w264) -> (w293:T8)
        n136 = Unbundle By Name(w293) -> ("Init Info.Bin Steps"=w292:i32, "Init Info.Base Resolution"=w267:dbl, "Init Info.nchannels"=w280:i32)
        n137 = for {
          N: w280 -> [_]
          tunnel: T2 {"Name"="", "Enable"=FALSE, "Offset"=0, "CFDLevel"=10, "ZeroX"=50, "dtcode"=0, "TrgLevel"=-100, "TrgEdge"=0} ("Channel") -> [w333]
          tunnel: [w332] -> w311 mode=indexing
          tunnel: [w322] -> w310 mode=indexing
          i -> [w322]
          # "Init values for Inp. Channels"
          n138 = Increment(x=w322) -> (x+1=w325:i32)
          n139 = Format Into String(format string="Ch.%d", w325) -> (resulting string=w323:string)  [unwired: 2 in, 1 out]
          n140 = Format Into String(format string="Inp.Chan %d", w325) -> (resulting string=w330:string)  [unwired: 2 in, 1 out]
          n141 = property on="HistoGraph" class="WFGraph (strict)"("Active Plot"=w322, "Plot.Plot Name"=w323) -> ()  [unwired: 2 in, 2 out]
          n142 = Bundle By Name(cluster=w333, "Name"=w330, "Enable"=TRUE, "Offset"=0, "CFDLevel"=-100 ("CFDZeroX"), "ZeroX"=-10 ("CFDLevel"), "dtcode"=0, "TrgLevel"=-100, "TrgEdge"=0) -> (w332:T2)
          n143 = property on="TTraceGraph" class="WFGraph (strict)"("Active Plot"=w322, "Plot.Plot Name"=w323) -> ()  [unwired: 2 in, 2 out]
        }
        n144 = Bundle By Name(cluster=T5 {"Histos"=[], "Cmd"=enum."_none_", "TimeTrace"=[], "Bin"=0, "Total bin"=0, "Status"="", "Resol"=0.0, "DeltaT"=0.0, "nChannels"=0} ("MH_GUIThread_QData"), "Cmd"=TH260_VisThread_QCmds."nChannels", "nChannels"=w280) -> (w282:T5)
        n145 = call "TH260_CalcBinningValues.vi"("BaseRes"=w267, "Bin Steps"=w292) -> ("BinningValues"=w297:cluster{"String":string, "Value":i32}[])  [unwired: 9 in]
        n146 = property on="Binning" class="Ring (strict)"("StringsAndValues[]"=w297) -> ()  [unwired: 2 in, 2 out]
        n147 = Bundle By Name(cluster=T7 {"Cmd"=enum."Proc", "nActual"=0, "Buffer"=[], "TickCount"=0, "Param"=0} ("MH_DataProcThread_QData"), "Param"=w280, "Cmd"=TH260_DataProcThread_QCmds."SetNumChannels") -> (w286:T7)
        n148 = Enqueue Element(queue=w279, element=w282) -> ()  [unwired: 2 in, 3 out]
        n149 = Enqueue Element(queue=w287, element=w286) -> ()  [unwired: 2 in, 3 out]
        n150 = local write "Channels"(w311) -> ()
        n151 = Bundle By Name(cluster=w293, "Channels"=w311, "CurrentChannels"=w310, "SyncDivider"=w307, "SyncOffset"=w306, "SyncZeroX"=w305, "SyncCFDLevel"=w304, "SyncTrgEdge"=w266, "SyncTrgLevel"=w265, "Binning"=w303, "HistoOffset"=w302, "AcqTime"=w301, "StopOvl."=w300, "OvlLevel"=w299, "StartMeas"=w298, "Run cont."=w296, "BitShift"=w278, "HistoAcqTime"=w277) -> (w289:T8)
        n152 = case shown="\"TimeHarp 260 P\"" w263 {
          tunnel: [FALSE TRUE] -> w262
          tunnel: [w315 w317] -> w260
          frame Default {
            w315 = T10[] [enum."SetSyncDivider", enum."SetSyncOffset", enum."SetSyncTrg", enum."SetInpChanEnable", enum."SetInpChanOffset", enum."SetInpChanTrg", enum."SetBinning", enum."SetHistoOffset", enum."Resize", enum."EnableControls", enum."GetRates", enum."SetBitShift", enum."SetHistoAcqTime", enum."WriteStatus"] items=["Idle", "Init", "SetInpChanEnable", "SetInpChanOffset", "SetInpChanCFD", "SetInpChanTrg", "SetInpChanDeadtime", "SetSyncDivider", "SetSyncCFD", "SetSyncTrg", "SetSyncOffset", "SetBinning", "SetHistoOffset", "SetHistoLen", "SetStopOvl", "SetBitShift", "SetHistoAcqTime", "GetRates", "StartMeas", "StopMeas", "AbortMeas", "GetResolution", "GetHisto", "ReadFiFo", "WriteStatus", "Resize", "EnableControls", "DisableControls", "Error", "Exit"]
          }
          frame "TimeHarp 260 P" {
            w317 = T10[] [enum."SetSyncDivider", enum."SetSyncOffset", enum."SetSyncCFD", enum."SetInpChanEnable", enum."SetInpChanOffset", enum."SetInpChanCFD", enum."SetInpChanDeadtime", enum."SetBinning", enum."SetHistoOffset", enum."Resize", enum."EnableControls", enum."GetRates", enum."SetBitShift", enum."SetHistoAcqTime", enum."WriteStatus"] items=["Idle", "Init", "SetInpChanEnable", "SetInpChanOffset", "SetInpChanCFD", "SetInpChanTrg", "SetInpChanDeadtime", "SetSyncDivider", "SetSyncCFD", "SetSyncTrg", "SetSyncOffset", "SetBinning", "SetHistoOffset", "SetHistoLen", "SetStopOvl", "SetBitShift", "SetHistoAcqTime", "GetRates", "StartMeas", "StopMeas", "AbortMeas", "GetResolution", "GetHisto", "ReadFiFo", "WriteStatus", "Resize", "EnableControls", "DisableControls", "Error", "Exit"]
          }
        }
        n153 = Not(x=w262) -> (.not. x?=w261:bool)
        n154 = property on="dtcode" class="Ring (strict)"("Visible"=w262) -> ()  [unwired: 2 in, 2 out]
        n155 = property on="SyncZeroX" class="DigNum (strict)"("Visible"=w262) -> ()  [unwired: 2 in, 2 out]
        n156 = property on="SyncCFDLevel" class="DigNum (strict)"("Visible"=w262) -> ()  [unwired: 2 in, 2 out]
        n157 = local write "Binning"(w303) -> ()
        n158 = local write "HistoOffset"(w302) -> ()
        n159 = local write "StopOvl."(w300) -> ()
        n160 = local write "OvlLevel"(w299) -> ()
        n161 = local write "Start"(w298) -> ()
        n162 = local write "Run continuously"(w296) -> ()
        n163 = local write "BitShift"(w278) -> ()
        n164 = local write "AcqTime"(w301) -> ()
        n165 = local write "HistoAcqTime"(w277) -> ()
        n166 = property on="CFDLevel" class="DigNum (strict)"("Visible"=w262) -> ()  [unwired: 2 in, 2 out]
        n167 = property on="ZeroX" class="DigNum (strict)"("Visible"=w262) -> ()  [unwired: 2 in, 2 out]
        n168 = property on="SyncTrgLevel" class="DigNum (strict)"("Visible"=w261) -> ()  [unwired: 2 in, 2 out]
        n169 = property on="SyncTrgEdge" class="Ring (strict)"("Visible"=w261) -> ()  [unwired: 2 in, 2 out]
        n170 = property on="TrgLevel" class="DigNum (strict)"("Visible"=w261) -> ()  [unwired: 2 in, 2 out]
        n171 = property on="TrgEdge" class="Ring (strict)"("Visible"=w261) -> ()  [unwired: 2 in, 2 out]
        n172 = Build Array (concatenate)(w309, w260) -> (w308:T10[])
      }
      frame "SetInpChanEnable" {
        n173 = Unbundle By Name(w340) -> ("DevIdx"=w339:i32, "Channels"=w334:T2[], "CurrentChannels"=w335:i32[])
        n174 = for {
          tunnel: w339 -> [w347]
          shift-right: [w346] -> w338
          shift-left: errorcluster {"status"=FALSE, "code"=0, "source"=""} ("error out") -> [w345]
          tunnel: w335 -> [w341] mode=indexing
          tunnel: w334 -> [w344]
          n175 = Index Array(array=w344, index=w341) -> (element=w343:T2)
          n176 = Unbundle By Name(w343) -> ("Enable"=w342:bool)
          n177 = call "TH260_SetInputChannelEnable.vi"("error in (no error)"=w345, "enable"=w342, "channel"=w341, "devidx"=w347) -> ("error out"=w346:errorcluster)  [unwired: 6 in, 1 out]
        }
      }
      frame "SetInpChanOffset" {
        n178 = Unbundle By Name(w354) -> ("DevIdx"=w353:i32, "Channels"=w348:T2[], "CurrentChannels"=w349:i32[])
        n179 = for {
          tunnel: w353 -> [w359]
          shift-right: [w356] -> w352
          shift-left: errorcluster {"status"=FALSE, "code"=0, "source"=""} ("error out") -> [w357]
          tunnel: w349 -> [w358] mode=indexing
          tunnel: w348 -> [w361]
          n180 = Index Array(array=w361, index=w358) -> (element=w360:T2)
          n181 = Unbundle By Name(w360) -> ("Offset"=w355:i32)
          n182 = call "TH260_SetInputChannelOffset.vi"("error in (no error)"=w357, "offset"=w355, "channel"=w358, "devidx"=w359) -> ("error out"=w356:errorcluster)  [unwired: 6 in, 1 out]
        }
      }
      frame "SetInpChanCFD" {
        n183 = Unbundle By Name(w368) -> ("DevIdx"=w367:i32, "Channels"=w362:T2[], "CurrentChannels"=w363:i32[])
        n184 = for {
          tunnel: w367 -> [w371]
          shift-right: [w373] -> w366
          shift-left: errorcluster {"status"=FALSE, "code"=0, "source"=""} ("error out") -> [w374]
          tunnel: w363 -> [w372] mode=indexing
          tunnel: w362 -> [w376]
          n185 = Index Array(array=w376, index=w372) -> (element=w375:T2)
          n186 = Unbundle By Name(w375) -> ("CFDLevel"=w370:i32, "ZeroX"=w369:i32)
          n187 = call "TH260_SetInputCFD.vi"("channel"=w372, "error in (no error)"=w374, "CFD ZeroCross"=w369, "CFD Level"=w370, "devidx"=w371) -> ("error out"=w373:errorcluster)  [unwired: 5 in, 1 out]
        }
      }
      frame "SetInpChanTrg" {
        n188 = Unbundle By Name(w383) -> ("DevIdx"=w382:i32, "Channels"=w377:T2[], "CurrentChannels"=w378:i32[])
        n189 = for {
          tunnel: w382 -> [w386]
          shift-right: [w388] -> w381
          shift-left: errorcluster {"status"=FALSE, "code"=0, "source"=""} ("error out") -> [w389]
          tunnel: w378 -> [w387] mode=indexing
          tunnel: w377 -> [w391]
          n190 = Index Array(array=w391, index=w387) -> (element=w390:T2)
          n191 = Unbundle By Name(w390) -> ("TrgLevel"=w385:i32, "TrgEdge"=w384:i32)
          n192 = call "TH260_SetInputEdgeTrg.vi"("channel"=w387, "error in (no error)"=w389, "edge"=w384, "level"=w385, "devidx"=w386) -> ("error out"=w388:errorcluster)  [unwired: 5 in, 1 out]
        }
      }
      frame "SetInpChanDeadtime" {
        n193 = Unbundle By Name(w398) -> ("DevIdx"=w397:i32, "Channels"=w392:T2[], "CurrentChannels"=w393:i32[])
        n194 = for {
          tunnel: w397 -> [w400]
          shift-right: [w402] -> w396
          shift-left: errorcluster {"status"=FALSE, "code"=0, "source"=""} ("error out") -> [w403]
          tunnel: w393 -> [w401] mode=indexing
          tunnel: w392 -> [w405]
          n195 = Index Array(array=w405, index=w401) -> (element=w404:T2)
          n196 = Unbundle By Name(w404) -> ("dtcode"=w399:i32)
          n197 = call "TH260_SetInputDeadTime.vi"("error in (no error)"=w403, "dtcode"=w399, "channel"=w401, "devidx"=w400) -> ("error out"=w402:errorcluster)  [unwired: 6 in, 1 out]
        }
      }
      frame "SetSyncDivider" {
        n198 = Unbundle By Name(w413) -> ("DevIdx"=w412:i32, "SyncDivider"=w408:i32)
        n199 = Power Of 2(x=w408) -> (2^x=w407:dbl)
        n200 = To Long Integer(number=w407) -> (32bit integer=w406:i32)
        n201 = call "TH260_SetSyncDiv.vi"("SyncDivider"=w406, "devidx"=w412) -> ("error out"=w410:errorcluster)  [unwired: 8 in, 1 out]
        n202 = flat-sequence {
          tunnel: w410 -> [w414]
          tunnel: [w414] -> w409
          frame #0 {
            n203 = Wait (ms)(milliseconds to wait=u32 100) -> ()  [unwired: 1 out]
          }
        }
      }
      frame "SetSyncTrg" {
        n204 = Unbundle By Name(w421) -> ("DevIdx"=w418:i32, "SyncTrgLevel"=w416:i32, "SyncTrgEdge"=w417:i32)
        n205 = call "TH260_SetSyncEdgeTrg.vi"("edge"=w417, "level"=w416, "devidx"=w418) -> ("error out"=w419:errorcluster)  [unwired: 7 in, 1 out]
      }
      frame "SetSyncCFD" {
        n206 = Unbundle By Name(w427) -> ("DevIdx"=w424:i32, "SyncCFDLevel"=w422:i32, "SyncZeroX"=w423:i32)
        n207 = call "TH260_SetSyncCFD.vi"("CFD ZeroCross"=w423, "CFD Level"=w422, "devidx"=w424) -> ("error out"=w425:errorcluster)  [unwired: 7 in, 1 out]
      }
      frame "SetSyncOffset" {
        n208 = Unbundle By Name(w432) -> ("DevIdx"=w430:i32, "SyncOffset"=w429:i32)
        n209 = call "TH260_SetSyncChannelOffset.vi"("Offset"=w429, "devidx"=w430) -> ("error out"=w431:errorcluster)  [unwired: 8 in, 1 out]
      }
      frame "SetBinning" {
        # "When binning is changed the new resolution is querried"
        n210 = Unbundle By Name(w439) -> ("DevIdx"=w437:i32, "Binning"=w436:i32)
        n211 = call "TH260_SetBinning.vi"("Binning"=w436, "devidx"=w437) -> ("error out"=w438:errorcluster)  [unwired: 8 in, 1 out]
        n212 = Build Array (concatenate)(TH260_UIThread_Cmds."GetResolution", w434) -> (w435:T10[])
      }
      frame "SetHistoOffset" {
        n213 = Unbundle By Name(w444) -> ("DevIdx"=w441:i32, "HistoOffset"=w440:i32)
        n214 = call "TH260_SetOffset.vi"("Offset"=w440, "devidx"=w441) -> ("error out"=w442:errorcluster)  [unwired: 8 in, 1 out]
      }
      frame "SetStopOvl" {
        n215 = Unbundle By Name(w450) -> ("DevIdx"=w447:i32, "StopOvl."=w446:bool, "OvlLevel"=w445:u32)
        n216 = call "TH260_SetStopOverflow.vi"("stopcount"=w445, "StopOnOverflow"=w446, "devidx"=w447) -> ("error out"=w448:errorcluster)  [unwired: 7 in, 1 out]
      }
      frame "SetBitShift" {
        n217 = Unbundle By Name(w454) -> ("BitShift"=w452:i32, "SyncRate"=w453:i32)
        n218 = Negate(x=w452) -> (-x=w462:i32)
        n219 = Bundle By Name(cluster=T7 {"Cmd"=enum."Proc", "nActual"=0, "Buffer"=[], "TickCount"=0, "Param"=0} ("MH_DataProcThread_QData"), "Param"=w462, "Cmd"=TH260_DataProcThread_QCmds."SetShift") -> (w468:T7)
        n220 = To Double Precision Float(number=w452) -> (double precision float=w467:dbl)
        n221 = To Double Precision Float(number=w453) -> (double precision float=w466:dbl)
        n222 = Power Of 2(x=w467) -> (2^x=w465:dbl)
        n223 = Enqueue Element(queue=w455, element=w468) -> ()  [unwired: 2 in, 3 out]
        n224 = Multiply(x=w465, y=1000.0) -> (x*y=w464:dbl)
        n225 = Divide(x=w464, y=w466) -> (x/y=w451:dbl)
        "DeltaT" <- w451
        n226 = Bundle By Name(cluster=T5 {"Histos"=[], "Cmd"=enum."_none_", "TimeTrace"=[], "Bin"=0, "Total bin"=0, "Status"="", "Resol"=0.0, "DeltaT"=0.0, "nChannels"=0} ("MH_GUIThread_QData"), "DeltaT"=w451, "Cmd"=TH260_VisThread_QCmds."DeltaT") -> (w463:T5)
        n227 = Enqueue Element(queue=w456, element=w463) -> ()  [unwired: 2 in, 3 out]
      }
      frame "SetHistoAcqTime" {
        n228 = Unbundle By Name(w471) -> ("SyncRate"=w477:i32, "HistoAcqTime"=w470:dbl)
        n229 = To Double Precision Float(number=w477) -> (double precision float=w480:dbl)
        n230 = Multiply(x=w480, y=w470) -> (x*y=w479:dbl)
        n231 = Round To Nearest(number=w479) -> (nearest integer value=w478:dbl)
        n232 = To Long Integer(number=w478) -> (32bit integer=w476:i32)
        n233 = Bundle By Name(cluster=T7 {"Cmd"=enum."Proc", "nActual"=0, "Buffer"=[], "TickCount"=0, "Param"=0} ("MH_DataProcThread_QData"), "Param"=w476, "Cmd"=TH260_DataProcThread_QCmds."SetHistAcqTime") -> (w475:T7)
        n234 = Enqueue Element(queue=w472, element=w475) -> ()  [unwired: 2 in, 3 out]
      }
      frame "GetRates" {
        n235 = Unbundle By Name(w484) -> ("Init Info.nchannels"=w491:i32, "Channels"=w485:T2[], "DevIdx"=w486:i32)
        n236 = call "TH260_GetSyncRate.vi"("devidx"=w486) -> ("error out"=w490:errorcluster, "rate"=w482:i32)  [unwired: 8 in, 1 out]
        n237 = Format Into String(format string="Sync Rate: %d cps\n", w482) -> (resulting string=→"SyncRate":string)  [unwired: 2 in, 1 out]
        n238 = for {
          N: w491 -> [_]
          tunnel: w486 -> [w499]
          tunnel: [w496] -> w488 mode=indexing
          shift-right: [w498] -> w492
          shift-left: w490 -> [w500]
          tunnel: w485 -> [w495] mode=indexing
          i -> [w497]
          n239 = Unbundle By Name(w495) -> ("Enable"=w494:bool)
          n240 = case shown="True" w494 {
            tunnel: w500 -> [w501 w506]
            tunnel: w499 -> [_ w505]
            tunnel: [w501 w504] -> w498
            tunnel: w497 -> [_ w503]
            tunnel: [_ w502] -> w496
            frame False {
            }
            frame True {
              n241 = call "TH260_GetCountRate.vi"("error in (no error)"=w506, "Channel"=w503, "devidx"=w505) -> ("error out"=w504:errorcluster, "rate"=w502:i32)  [unwired: 6 in, 1 out]
            }
          }
        }
        "CountRates" <- w488
        n242 = Bundle By Name(cluster=w484, "SyncRate"=w482) -> (w483:T8)
      }
      frame "StartMeas" {
        n243 = Bundle By Name(cluster=T7 {"Cmd"=enum."Proc", "nActual"=0, "Buffer"=[], "TickCount"=0, "Param"=0} ("MH_DataProcThread_QData"), "Cmd"=TH260_DataProcThread_QCmds."Init") -> (w508:T7)
        n244 = Unbundle By Name(w517) -> ("DevIdx"=w515:i32, "AcqTime"=w511:i32)
        n245 = Enqueue Element(queue=w510, element=w508) -> ()  [unwired: 2 in, 3 out]
        n246 = call "TH260_StartMeas.vi"("Acquisition time"=w511, "devidx"=w515) -> ("error out"=w516:errorcluster)  [unwired: 8 in, 1 out]
        n247 = Build Array (concatenate)(w514, TH260_UIThread_Cmds."ReadFiFo") -> (w513:T10[])
      }
      frame "StopMeas" {
        n248 = Unbundle By Name(w523) -> ("Run cont."=w518:bool, "DevIdx"=w524:i32)
        n249 = call "TH260_StopMeas.vi"("devidx"=w524) -> ("error out"=w525:errorcluster)  [unwired: 9 in, 1 out]
        n250 = case shown="True" w518 {
          tunnel: w523 -> [w529 w531]
          tunnel: [w528 w531] -> w522
          tunnel: [w526 w530] -> w521
          frame False {
            w526 = T10[] [enum."ReadFiFo"] items=["Idle", "Init", "SetInpChanEnable", "SetInpChanOffset", "SetInpChanCFD", "SetInpChanTrg", "SetInpChanDeadtime", "SetSyncDivider", "SetSyncCFD", "SetSyncTrg", "SetSyncOffset", "SetBinning", "SetHistoOffset", "SetHistoLen", "SetStopOvl", "SetBitShift", "SetHistoAcqTime", "GetRates", "StartMeas", "StopMeas", "AbortMeas", "GetResolution", "GetHisto", "ReadFiFo", "WriteStatus", "Resize", "EnableControls", "DisableControls", "Error", "Exit"]
            w527 = FALSE ("StartMeas")
            n251 = Bundle By Name(cluster=w529, "StartMeas"=w527) -> (w528:T8)
            n252 = local write "Start"(w527) -> ()
          }
          frame True {
            w530 = T10[] [enum."ReadFiFo", enum."StartMeas"] items=["Idle", "Init", "SetInpChanEnable", "SetInpChanOffset", "SetInpChanCFD", "SetInpChanTrg", "SetInpChanDeadtime", "SetSyncDivider", "SetSyncCFD", "SetSyncTrg", "SetSyncOffset", "SetBinning", "SetHistoOffset", "SetHistoLen", "SetStopOvl", "SetBitShift", "SetHistoAcqTime", "GetRates", "StartMeas", "StopMeas", "AbortMeas", "GetResolution", "GetHisto", "ReadFiFo", "WriteStatus", "Resize", "EnableControls", "DisableControls", "Error", "Exit"]
          }
        }
        n253 = Build Array (concatenate)(w520, w521) -> (w519:T10[])
      }
      frame "AbortMeas" {
        w533 = FALSE ("StartMeas")
        n254 = Unbundle By Name(w535) -> ("DevIdx"=w536:i32)
        n255 = call "TH260_StopMeas.vi"("devidx"=w536) -> ("error out"=w537:errorcluster)  [unwired: 9 in, 1 out]
        n256 = Bundle By Name(cluster=w535, "StartMeas"=w533) -> (w534:T8)
        n257 = local write "Start"(w533) -> ()
      }
      frame "GetResolution" {
        # "Resolution in ns"
        # "Gets resolution in ps"
        # "Resolution is saved in UIThread Data cluster in ns"
        n258 = Unbundle By Name(w546) -> ("DevIdx"=w548:i32)
        n259 = call "TH260_GetResolution.vi"("devidx"=w548) -> ("error out"=w547:errorcluster, "resolution"=w544:dbl)  [unwired: 8 in, 1 out]
        n260 = Divide(x=w544, y=1000.0) -> (x/y=w540:dbl)
        n261 = Bundle By Name(cluster=w546, "Resolution"=w540) -> (w545:T8)
        n262 = Bundle By Name(cluster=T5 {"Histos"=[], "Cmd"=enum."_none_", "TimeTrace"=[], "Bin"=0, "Total bin"=0, "Status"="", "Resol"=0.0, "DeltaT"=0.0, "nChannels"=0} ("MH_GUIThread_QData"), "Resol"=w540, "Cmd"=TH260_VisThread_QCmds."Resol") -> (w538:T5)
        n263 = Enqueue Element(queue=w542, element=w538) -> ()  [unwired: 2 in, 3 out]
      }
      frame "ReadFiFo" {
        w558 = 2  # FLAG_FIFOFULL
        # "Reads photon records from HW and transferes them to DataProcThread via Queue."
        n264 = Unbundle By Name(w560) -> ("DevIdx"=w554:i32)
        n265 = call "TH260_GetFlags.vi"("devidx"=w554) -> ("error out"=w556:errorcluster, "flags"=w557:i32)  [unwired: 8 in, 1 out]
        n266 = And(x=w557, y=w558) -> (x .and. y?=w559:i32)
        n267 = Not Equal To 0?(x=w559) -> (x != 0?=w553:bool)
        "OverRun" <- w553
        n268 = case shown="False" w553 {
          tunnel: w556 -> [w570 w573]
          tunnel: [w569 w573] -> w555
          tunnel: w554 -> [w562 _]
          tunnel: w552 -> [w568 _]
          tunnel: w551 -> [w567 _]
          tunnel: [w567 w571] -> w550
          frame False {
            n269 = call "TH260_ReadFiFo.vi"("error in (no error)"=w570, "devidx"=w562) -> ("error out"=w569:errorcluster, "nactual"=w561:i32, "buffer"=w565:u32[])  [unwired: 6 in, 1 out]
            n270 = Bundle By Name(cluster=T7 {"Cmd"=enum."Proc", "nActual"=0, "Buffer"=[], "TickCount"=0, "Param"=0} ("MH_DataProcThread_QData"), "Buffer"=w565, "nActual"=w561, "Cmd"=TH260_DataProcThread_QCmds."Proc") -> (w563:T7)
            n271 = Enqueue Element(queue=w568, element=w563) -> ()  [unwired: 2 in, 3 out]
          }
          frame True {
            n272 = Build Array(TH260_UIThread_Cmds."AbortMeas") -> (w571:T10[])
          }
        }
      }
      frame "WriteStatus" {
        n273 = Unbundle By Name(w575) -> ("Status"=→"Status":string)
      }
      frame "Resize" {
        n274 = property on="Pane 3" class="Pane"() -> ("Width"=w582:u32)  [unwired: 2 in, 2 out]
        n275 = Subtract(x=w582, y=i16 100 ("b")) -> (x-y=w588:u32)
        n276 = Unbundle By Name(w577) -> ("Init Info.nchannels"=w585:i32)
        n277 = Quotient & Remainder(x=w588, y=i16 99 ("m")) -> (floor(x/y)=w587:u32)  [unwired: 1 out]
        n278 = In Range and Coerce(upper limit=w585, x=w587, lower limit=4) -> (coerced(x)=w586:u32)  [unwired: 1 out]
        n279 = Equal?(x=w585, y=w586) -> (x = y?=w584:bool)
        n280 = Not(x=w584) -> (.not. x?=w583:bool)
        n281 = property on="Channels" class="Arr (strict)"("HorizScroll"=w583, "Number of Columns"=w586, "Index Values"=u32[] [0]) -> ()  [unwired: 2 in, 2 out]
      }
      frame "EnableControls" {
        n282 = property class="VI"() -> ("Panel"=w593:refnum<vi>)  [unwired: 2 in, 2 out]
        n283 = property class="Pnl"(reference=w593) -> ("Controls[]"=w592:refnum<vi>[])  [unwired: 1 in, 2 out]
        n284 = property class="Pnl"(reference=w593) -> ("Decos[]"=w594:refnum<vi>[])  [unwired: 1 in, 2 out]
        n285 = for {
          tunnel: w594 -> [w598] mode=indexing
          tunnel: TRUE -> [w597]
          n286 = property class="Decor"(reference=w598, "Visible"=w597) -> ()  [unwired: 1 in, 2 out]
        }
        n287 = for {
          tunnel: w592 -> [w601] mode=indexing
          tunnel: T11."Enabled" ("Disabled") -> [w600]
          tunnel: [w599] -> _
          n288 = property class="Ctl"(reference=w601, "DisabledEnum"=w600) -> (error out=w599:errorcluster)  [unwired: 1 in, 1 out]
        }
      }
      frame "DisableControls" {
        n289 = property class="VI"() -> ("Panel"=w605:refnum<vi>)  [unwired: 2 in, 2 out]
        n290 = property class="Pnl"(reference=w605) -> ("Controls[]"=w604:refnum<vi>[])  [unwired: 1 in, 2 out]
        n291 = property class="Pnl"(reference=w605) -> ("Decos[]"=w606:refnum<vi>[])  [unwired: 1 in, 2 out]
        n292 = for {
          tunnel: w606 -> [w610] mode=indexing
          tunnel: FALSE -> [w609]
          n293 = property class="Decor"(reference=w610, "Visible"=w609) -> ()  [unwired: 1 in, 2 out]
        }
        n294 = for {
          tunnel: w604 -> [w613] mode=indexing
          tunnel: T11."Disabled and Grayed Out" ("Disabled") -> [w612]
          tunnel: [w611] -> _
          n295 = property class="Ctl"(reference=w613, "DisabledEnum"=w612) -> (error out=w611:errorcluster)  [unwired: 1 in, 1 out]
        }
      }
      frame "Error" {
        w614 = T10[] [enum."Exit"] items=["Idle", "Init", "SetInpChanEnable", "SetInpChanOffset", "SetInpChanCFD", "SetInpChanTrg", "SetInpChanDeadtime", "SetSyncDivider", "SetSyncCFD", "SetSyncTrg", "SetSyncOffset", "SetBinning", "SetHistoOffset", "SetHistoLen", "SetStopOvl", "SetBitShift", "SetHistoAcqTime", "GetRates", "StartMeas", "StopMeas", "AbortMeas", "GetResolution", "GetHisto", "ReadFiFo", "WriteStatus", "Resize", "EnableControls", "DisableControls", "Error", "Exit"]
        w617 = T14 1 items=["no dialog", "OK message", "continue or stop message", "OK message + warnings", "continue/stop + warnings"] ("type of dialog (OK msg:1)")
        # "Error case: If an error occures the user is informed and the programm terminates. Add your own code to handle error events (e.g. exception lists, etc.)"
        n296 = call <vilib>:"Simple Error Handler.vi"("type of dialog (OK msg:1)"=w617, "error in (no error)"=w616) -> ()  [unwired: 3 in, 5 out]
      }
      frame "Exit" {
        n297 = Release Queue(queue=w619) -> ()  [unwired: 2 in, 3 out]
        n298 = Release Queue(queue=w618) -> ()  [unwired: 2 in, 3 out]
        n299 = Unbundle By Name(w623) -> ("DevIdx"=w622:i32)
        n300 = call "TH260_CloseDevice.vi"("devidx"=w622) -> ("error out"=w621:errorcluster)  [unwired: 9 in, 1 out]
      }
    }
    n301 = call "TH260_EnQError.vi"("error in (no error)"=w24, "Cmds_in"=w22) -> ("error out"=w23:errorcluster, "Cmds_out"=w21:T10[])  [unwired: 8 in]
  }
  n302 = call "TH260_DataProcThread.vi"("TH260_VisThread_QRef"=w7, "TH260_DataProcThread_QRef"=w1) -> ()  [unwired: 10 in]
  n303 = while {
    tunnel: w7 -> [w632]
    shift-right: [w628] -> _
    shift-left: T4 {"Resol"=0.0, "DeltaT"=0.0, "NumChannels"=0} -> [w629]
    tunnel: w1 -> [w627]
    stop <- w625 stop-if-true
    # "VisualizationThread"
    n304 = Dequeue Element(queue=w632, timeout in ms (-1)=100) -> (element=w630:T5, error out=w625:errorcluster)  [unwired: 1 in, 2 out]
    n305 = Unbundle By Name(w630) -> ("Cmd"=w631:T6)
    n306 = case shown="\"Histo\"" w631 {
      tunnel: w630 -> [_ w645 w647 w659 w667 w671 w675]
      tunnel: w629 -> [w635 w643 w649 w651 w666 w670 w674]
      tunnel: [w635 w643 w648 w651 w666 w669 w673] -> w628
      tunnel: w627 -> [w634 _ _ _ w663 _ _]
      tunnel: w625 -> [w633 _ _ _ _ _ _]
      frame "_none_", Default {
        n307 = case shown="No Error" w633 {
          tunnel: w634 -> [w639 _]
          frame No Error {
            n308 = Get Queue Status(queue=w639) -> (# elements in queue=w637:i32)  [unwired: 2 in, 7 out]
            n309 = Format Into String(format string="Elements in Q: %d", w637) -> (resulting string=w636:string)  [unwired: 2 in, 1 out]
            n310 = local write "Status"(w636) -> ()
          }
          frame Error {
          }
        }
      }
      frame "Histo" {
        n311 = Unbundle By Name(w645) -> ("Histos"=w640:u32[][])
        n312 = Unbundle By Name(w643) -> ("Resol"=w642:dbl)
        n313 = Bundle(0.0, "Resol"=w642, "Histos"=w640) -> (→"HistoGraph":cluster{dbl, "Resol":dbl, "Histos":u32[][]})  [unwired: 1 in]
      }
      frame "nChannels" {
        n314 = Unbundle By Name(w647) -> ("nChannels"=w646:i32)
        n315 = Bundle By Name(cluster=w649, "NumChannels"=w646) -> (w648:T4)
      }
      frame "TTrace" {
        n316 = Unbundle By Name(w659) -> ("Total bin"=w658:u64, "Bin"=w657:i32, "TimeTrace"=w656:u32[][])
        n317 = Unbundle By Name(w651) -> ("DeltaT"=w650:dbl)
        n318 = call "TH260_TTraceToGraph.vi"("DeltaT"=w650, "TimeTrace"=w656, "Bin"=w657, "Total bin"=w658) -> ("TimeTrace_out"=w653:u32[][], "dt"=w654:dbl, "T0"=w655:dbl)  [unwired: 5 in]
        n319 = Bundle("T0"=w655, "dt"=w654, "TimeTrace_out"=w653) -> (→"TTraceGraph":T15)  [unwired: 1 in]
      }
      frame "Status" {
        n320 = Unbundle By Name(w667) -> ("Status"=w664:string)
        n321 = Get Queue Status(queue=w663) -> (# elements in queue=w662:i32)  [unwired: 2 in, 7 out]
        n322 = Format Into String(format string="\t\tElements in Q: %d", w662) -> (resulting string=w660:string)  [unwired: 2 in, 1 out]
        n323 = Concatenate Strings(w664, w660) -> (w665:string)
        n324 = local write "Status"(w665) -> ()
      }
      frame "DeltaT" {
        n325 = Unbundle By Name(w671) -> ("DeltaT"=w668:dbl)
        n326 = Bundle By Name(cluster=w670, "DeltaT"=w668) -> (w669:T4)
      }
      frame "Resol" {
        n327 = Unbundle By Name(w675) -> ("Resol"=w672:dbl)
        n328 = Bundle By Name(cluster=w674, "Resol"=w672) -> (w673:T4)
      }
    }
  }
